vi "Force To Current.vi"(8 "error in (no error)":errorcluster, 9 "Pressure Servo Settings":T1={"Center Point"=2.5, "Area"=0.004536, "PA to PSI"=0.000145038, "Off Value"=0.004536} {"Off Value" format="%.3f"; "PA to PSI" format="%.9f"; "Area" format="%.9f"; "Center Point" format="%.3f"}, 10 "Force":dbl[unit], 11 "Force To Turbo Valve Current in":refnum<class "Force To Turbo Valve Current.lvclass">) -> (0 "error out":errorcluster, 2 "Current":dbl, 3 "Force To Turbo Valve Current out":refnum<class "Force To Turbo Valve Current.lvclass">)   [LabVIEW 2015, in "Force To Turbo Valve Current.lvclass"]
uses:
  Force To Turbo Valve Current.lvclass
  Typedefs/Pressure Servo Valve Settings.ctl
  Typedefs/FAMT Typedefs.lvlib
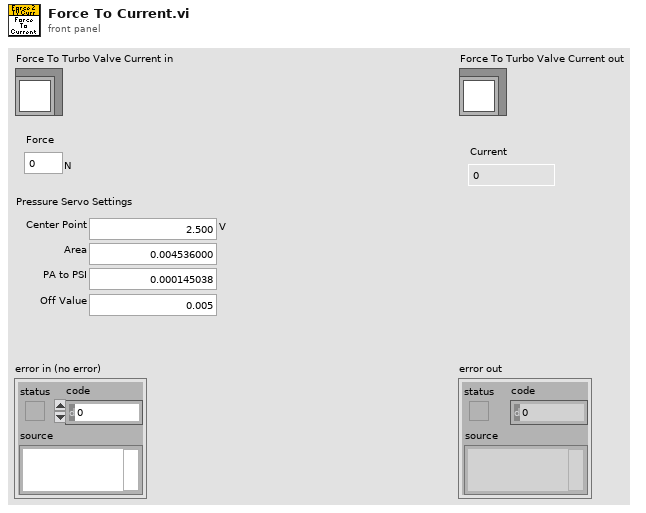
[diagram p1: front panel]
types:
  T1 = typedef "FAMT Typedefs.lvlib/Pressure Servo Valve Settings.ctl" = cluster{"Center Point":dbl[unit], "Area":dbl, "PA to PSI":dbl, "Off Value":dbl}
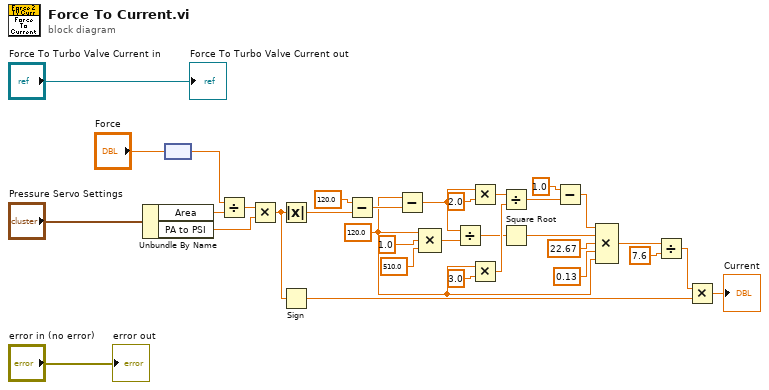
[diagram p0: block diagram]
diagram:
  w2 = 120.0 ("y")
  n1 = Unbundle By Name("Pressure Servo Settings") -> ("Area"=w32:dbl, "PA to PSI"=w30:dbl)
  n2 = node("Force") -> (w26:dbl)
  n3 = Divide(x=w26, y=w32) -> (x/y=w31:dbl)
  n4 = Multiply(x=w31, y=w30) -> (x*y=w5:dbl)
  n5 = Absolute Value(x=w5) -> (abs(x)=w29:dbl)
  n6 = Sign(1:w5) -> (0:w4:dbl)
  n7 = Subtract(x=120.0, y=w29) -> (x-y=w3:dbl)
  n8 = Subtract(x=w2, y=w3) -> (x-y=w18:dbl)
  n9 = Compound Arithmetic op=MULTIPLY(w2, 1.0 ("value"), 510.0 ("value")) -> (w19:dbl)
  n10 = Divide(x=w18, y=w19) -> (x/y=w14:dbl)
  n11 = Multiply(x=w18, y=2.0) -> (x*y=w22:dbl)
  n12 = Multiply(x=w2, y=3.0) -> (x*y=w23:dbl)
  n13 = Divide(x=w22, y=w23) -> (x/y=w17:dbl)
  n14 = Square Root(x=w14) -> (sqrt(x)=w1:dbl)
  n15 = Subtract(x=1.0, y=w17) -> (x-y=w15:dbl)
  n16 = Compound Arithmetic op=MULTIPLY(w15, w1, 22.67 ("value"), 0.13 ("value"), w2) -> (w11:dbl)
  n17 = Divide(x=w11, y=7.6) -> (x/y=w9:dbl)
  n18 = Multiply(x=w9, y=w4) -> (x*y=→"Current":dbl)
  "error out" <- "error in (no error)"
  "Force To Turbo Valve Current out" <- "Force To Turbo Valve Current in"
